vi "GEA2 Board ID to Board Index.vi"(0 "Board ID":string, 11 "Error In":errorcluster) -> (4 "Board Found?":bool, 6 "Report Text":string="Board not found.", 8 "Board Index":i32=-1, 10 "Boards Found":string[](array[string]), 15 "Error Out":errorcluster)   [LabVIEW 2023, in "GEA2_Toolkit.lvlib"]
doc: "This VI should be placed before the GEA2 Initialize VI. This VI will output the corresponding GEA2 bus index for a given NewFI board ID input."
uses:
  library/GEA2_Toolkit.lvlib
  C:/TechnologyLab/NI-2010/Drivers/GEA3 Toolkit/GEA3 DLL Source/GeaCommunication.dll
  GEA3 DLL Source/GeaCommunication.dll
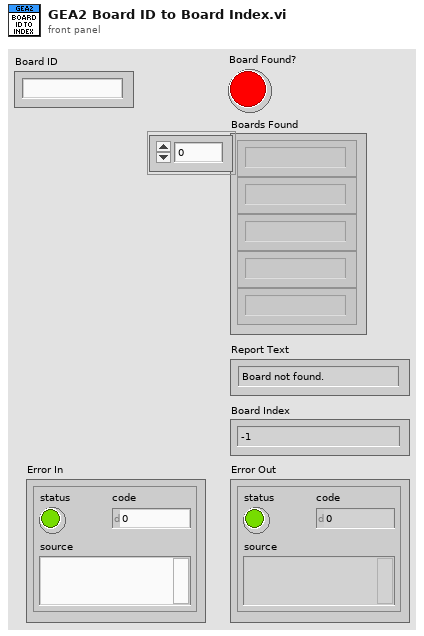
[diagram p1: front panel]
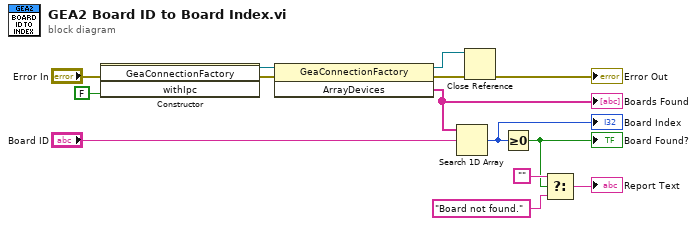
[diagram p0: block diagram]
diagram:
  n1 = constructor class="GeaConnectionFactory"(error in="Error In", "withIpc"=FALSE) -> (reference out=w14:refnum<k24>, error out=w13:errorcluster)  [unwired: 2 in, 2 out]
  n2 = invoke class="GeaConnectionFactory" method="ArrayDevices"(reference=w14, error in=w13) -> (reference out=w11:refnum<k24>, error out=w2:errorcluster, "ArrayDevices"=w3:string[])  [unwired: 1 in]
  "Boards Found" <- w3
  n3 = Search 1D Array(1D array=w3, element="Board ID") -> (index of element=w5:i32)  [unwired: 1 in]
  "Board Index" <- w5
  n4 = Close Reference(reference=w11, error in (no error)=w2) -> (error out=→"Error Out":errorcluster)
  n5 = Greater Or Equal To 0?(x=w5) -> (x >= 0?=w4:bool)
  "Board Found?" <- w4
  n6 = Select(t="", s=w4, f="Board not found.") -> (s? t:f=→"Report Text":string)
